vi "Programacion 13 Lester Roche.vi"() -> ()   [LabVIEW 2011]
panel:
  in  "Stop":bool
  out "Velocidad":dbl(knob) scale=0.0..180.0
  in  "Reducir":bool
  in  "Aumentar":bool
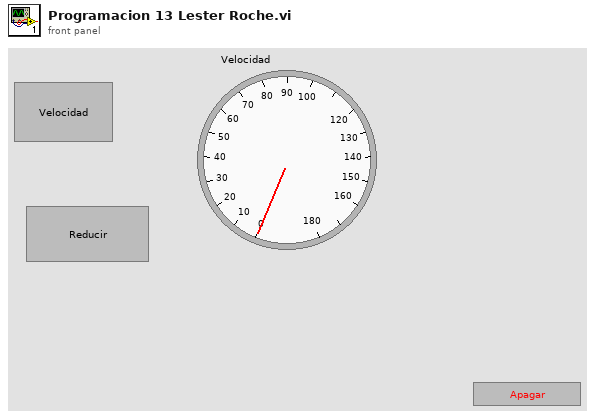
[diagram p1: front panel]
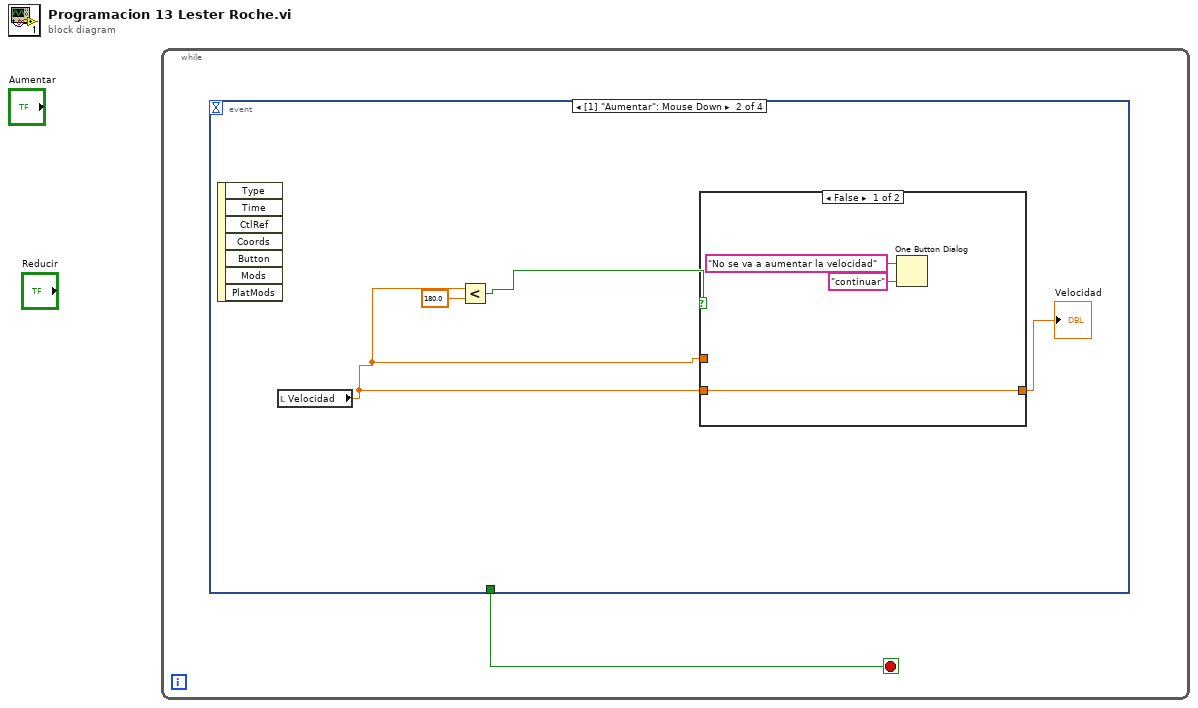
[diagram p0: block diagram]
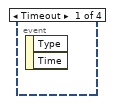
[diagram p2: hidden frame]
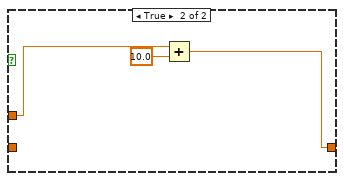
[diagram p3: hidden frame]
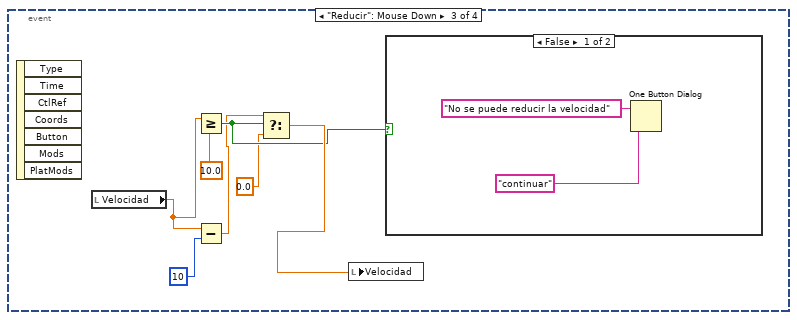
[diagram p4: hidden frame]
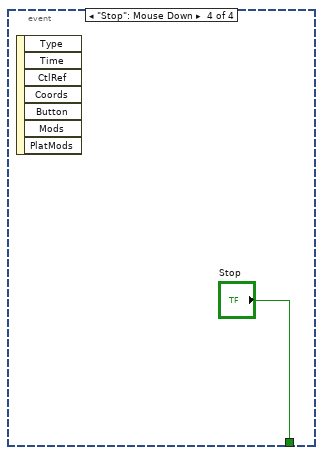
[diagram p6: hidden frame]
diagram:
  n1 = while {
    stop <- w1 stop-if-true
    n2 = event shown="[1] \"Aumentar\": Mouse Down" {
      selector: _ -> [_ _ _ _]
      dyn-events: _ -> [_ _ _ _]
      timeout: _ -> [_ _ _ _]
      tunnel: [_ _ _ "Stop"] -> w1
      event Timeout {
        n3 = event-data() -> ()  [unwired: 1 in, 2 out]
      }
      event "Aumentar": Mouse Down {
        n4 = event-data() -> ()  [unwired: 1 in, 7 out]
        n5 = local read "Velocidad"() -> (w2:dbl)
        n6 = Less?(x=w2, y=180.0) -> (x < y?=w4:bool)
        n7 = case shown="False" w4 {
          tunnel: [w6 w9] -> w3
          tunnel: w2 -> [w6 _]
          tunnel: w2 -> [_ w11]
          frame False {
            n8 = One Button Dialog(message="No se va a aumentar la velocidad", button name ("OK")="continuar") -> ()  [unwired: 1 out]
          }
          frame True {
            n9 = Add(x=w11, y=10.0) -> (x+y=w9:dbl)
          }
        }
        "Velocidad" <- w3
      }
      event "Reducir": Mouse Down {
        n10 = event-data() -> ()  [unwired: 1 in, 7 out]
        n11 = local read "Velocidad"() -> (w17:dbl)
        n12 = Greater Or Equal?(x=w17, y=10.0) -> (x >= y?=w14:bool)
        n13 = Subtract(x=w17, y=10) -> (x-y=w12:dbl)
        n14 = Select(t=w12, s=w14, f=0.0 ("t")) -> (s? t:f=w15:dbl)
        n15 = local write "Velocidad"(w15) -> ()
        n16 = case shown="False" w14 {
          frame False {
            n17 = One Button Dialog(message="No se puede reducir la velocidad", button name ("OK")="continuar") -> ()  [unwired: 1 out]
          }
          frame True {
          }
        }
      }
      event "Stop": Mouse Down {
        n18 = event-data() -> ()  [unwired: 1 in, 7 out]
      }
    }
  }
